vi "PH_Cam_BaseClass.panel.vi"(0 "object ref":refnum<vi>, 5 "error in (no error)":errorcluster) -> (19 "error out":errorcluster)   [LabVIEW 2014, in "PH_Cam_BaseClass.lvlib"]
doc: "This VI is the GUI to control a IEEE1394 Cam.\n\nLicense Agreement for this software:\n\nCopyright (C)\nGesellschaft für Schwerionenforschung, GSI\nPlanckstr. 1\n64291 Darmstadt\nGermany\n\nContact: D.Beck@gsi.de \n\nThis program is free software; you can redistribute it and/or modify it under the terms of the GNU General Public License as published by the Free Software Foundation; either version 2 of the license, or (at your option) any later version.\n\nThis program is distributed in the hope that it will be useful, but WITHOUT ANYW ARRANTY; without even the implied warranty of MERCHANTABILITY or FITNESS FOR A PARTICULAR PURPOSE. See the GNU General License for more details (http://www.gnu.org).\n\nGesellschaft für Schwerionenforschung, GSI\nPlanckstr. 1, 64291 Darmstadt, Germany\nFor all questions and ideas contact: M.Richter@gsi.de, H.Brand@gsi.de or D.Beck@gsi.de.\nLast update: 18-DEC-2002"
uses:
  PH_Cam_BaseClass.lvlib
  PH_StatusHandler/PH_StatusHandler.GUI element.ctl
  PH_Cam_BaseClass.GUI Refs.ctl
  CS_Core/CSObj/CSObj.lvlib
  CS_Core/CSSystem/CSSystemLib/CSSystemLib.lvlib
  PH_Common/PH_Common.lvlib
  PH_Class/PH_Class.lvlib
  PH_StatusHandler/PH_StatusHandler.lvlib
panel:
  out "PSDB Status":u32(colorbox)=6618880 caption="PSDB"
  out "Camera Status":T1 caption="Camera"
  in  "Tab Control":T2(tab)
  in  "Start Cam":bool
  in  "Get Histogram":bool
  in  "Logarithmic":bool
  out "Histogram":u32[](graph)
  in  "Save Image":bool
  in  "Show Image":bool
  in  "Palette":i32(ring) items=["Grey", "Binary", "Gradient", "Rainbow", "Temperature", "HMH"]
  in  "Scale Factor":i32=50 caption="%" min=30 max=500
  in  "Center of Gravity":bool
  in  "Subtract Background":bool
  in  "Center Cross":bool
  in  "Cam List":u32(ring)
  out "Cam Error":errorcluster
  out "Frames per second":dbl(knob) scale=0.0..30.0 scale format="%.1f"
  in  "Get Frame Rate":bool
  in  "Delete":bool
  in  "Exit":bool
  out "loop counter":i32
  # "PCS"
  # "3.40"
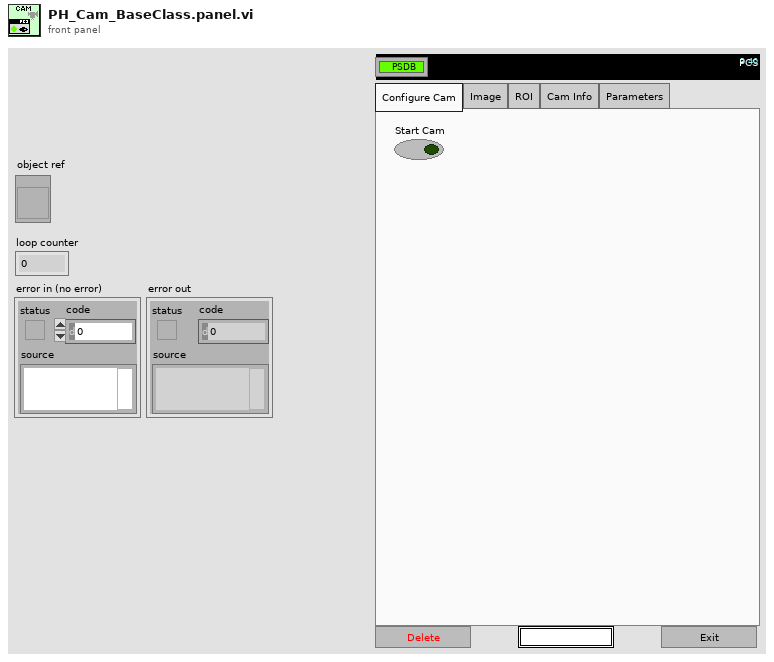
[diagram p1: front panel]
types:
  T1 = typedef "PH_StatusHandler.lvlib/PH_StatusHandler.GUI element.ctl" = u16
  T2 = enum32{"Configure Cam", "Image", "ROI", "Cam Info", "Parameters"}
  T3 = typedef "PH_Cam_BaseClass.lvlib/PH_Cam_BaseClass.GUI Refs.ctl" = cluster{"Frame Rate":refnum<vi>, "Get Frame Rate":refnum<vi>, "Show Image":refnum<vi>, "Get Histogram":refnum<vi>, "Mapping":refnum<vi>, "Histogram":refnum<vi>, "Center Cross":refnum<vi>, "Center of Gravity":refnum<vi>, "Scale Factor [%]":refnum<vi>, "Save Image":refnum<vi>, "Palette":refnum<vi>, "Subtract Background":refnum<vi>, "Cam Error":refnum<vi>, "On":refnum<vi>, "Cam List":refnum<vi>}
  T4 = cluster{"Cam Base ClassGui Refs":T3, "PSDB Status":refnum<vi>, "Status":refnum<vi>}
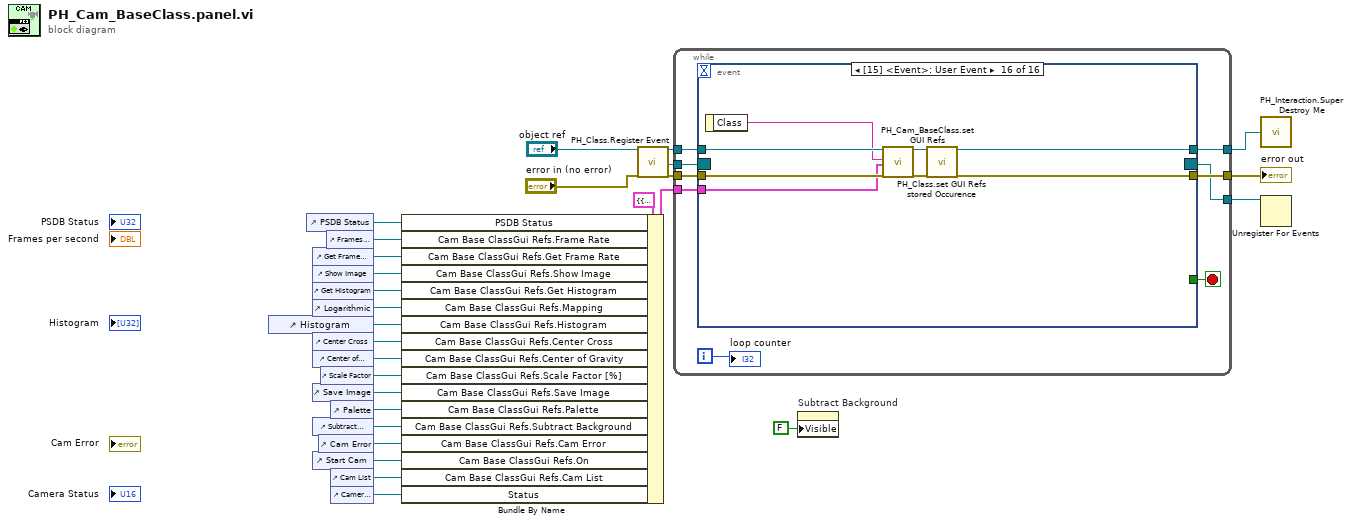
[diagram p0: block diagram]
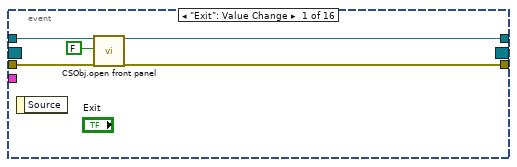
[diagram p2: hidden frame]
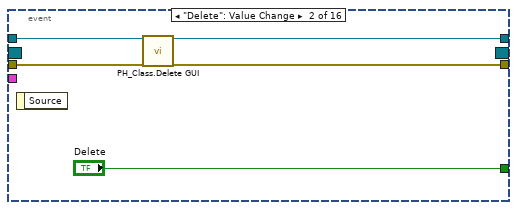
[diagram p3: hidden frame]
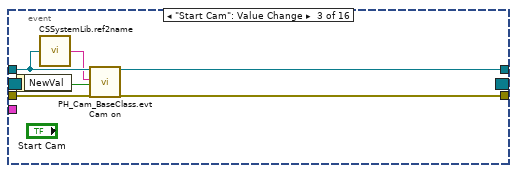
[diagram p4: hidden frame]
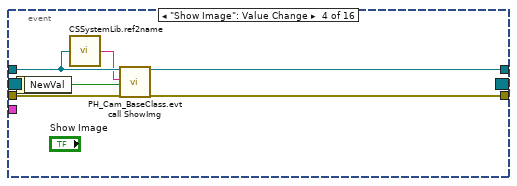
[diagram p5: hidden frame]
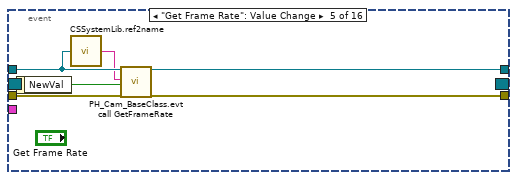
[diagram p6: hidden frame]
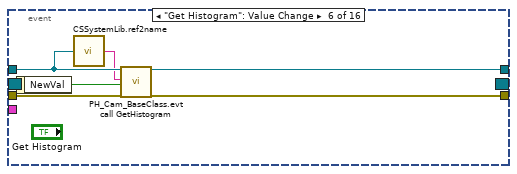
[diagram p7: hidden frame]
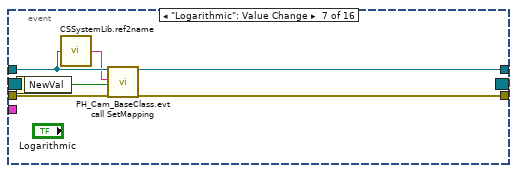
[diagram p8: hidden frame]
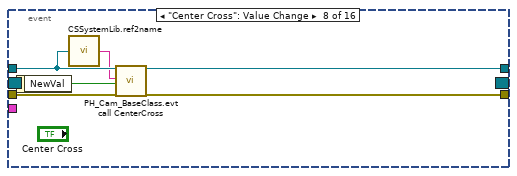
[diagram p9: hidden frame]
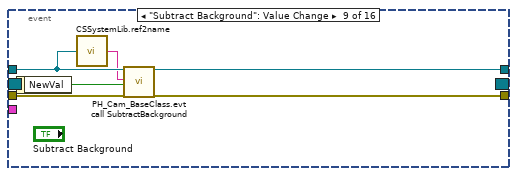
[diagram p10: hidden frame]
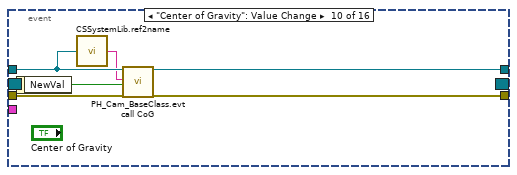
[diagram p11: hidden frame]
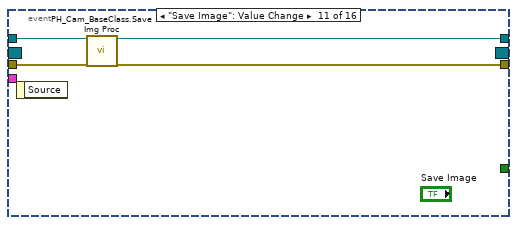
[diagram p12: hidden frame]
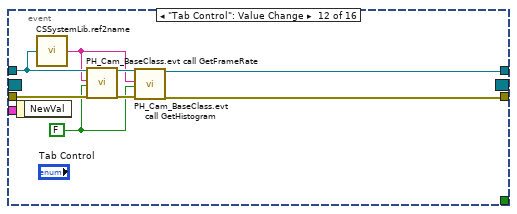
[diagram p13: hidden frame]
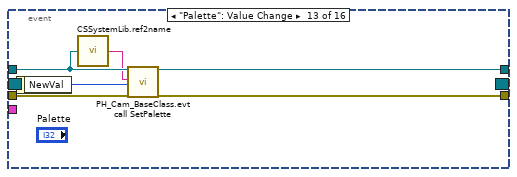
[diagram p14: hidden frame]
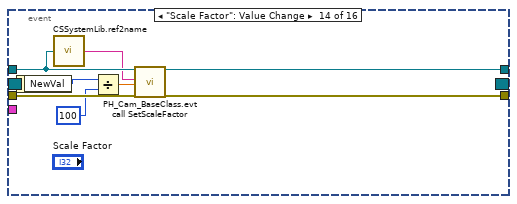
[diagram p15: hidden frame]
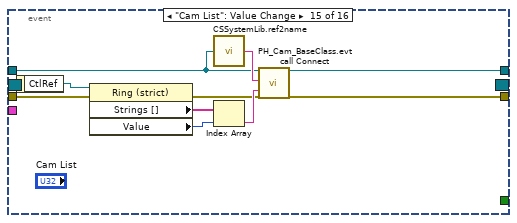
[diagram p16: hidden frame]
diagram:
  n1 = control-ref of="Histogram"() -> (w23:refnum<vi>)
  n2 = control-ref of="PSDB Status"() -> (w4:refnum<vi>)
  n3 = control-ref of="Get Frame Rate"() -> (w27:refnum<vi>)
  n4 = control-ref of="Show Image"() -> (w26:refnum<vi>)
  n5 = control-ref of="Get Histogram"() -> (w25:refnum<vi>)
  n6 = control-ref of="Logarithmic"() -> (w24:refnum<vi>)
  n7 = control-ref of="Center Cross"() -> (w16:refnum<vi>)
  n8 = control-ref of="Center of Gravity"() -> (w19:refnum<vi>)
  n9 = control-ref of="Save Image"() -> (w22:refnum<vi>)
  n10 = control-ref of="Subtract Background"() -> (w15:refnum<vi>)
  n11 = control-ref of="Start Cam"() -> (w12:refnum<vi>)
  n12 = control-ref of="Cam Error"() -> (w13:refnum<vi>)
  n13 = control-ref of="Scale Factor"() -> (w20:refnum<vi>)
  n14 = control-ref of="Frames per second"() -> (w28:refnum<vi>)
  n15 = control-ref of="Palette"() -> (w21:refnum<vi>)
  n16 = control-ref of="Cam List"() -> (w11:refnum<vi>)
  n17 = control-ref of="Camera Status"() -> (w1:refnum<vi>)
  n18 = Bundle By Name(cluster=T4 {"Cam Base ClassGui Refs"={"Frame Rate"=refnum, "Get Frame Rate"=refnum, "Show Image"=refnum, "Get Histogram"=refnum, "Mapping"=refnum, "Histogram"=refnum, "Center Cross"=refnum, "Center of Gravity"=refnum, "Scale Factor [%]"=refnum, "Save Image"=refnum, "Palette"=refnum, "Subtract Background"=refnum, "Cam Error"=refnum, "On"=refnum, "Cam List"=refnum}, "PSDB Status"=refnum, "Status"=refnum} ("GUI Refs to set"), "PSDB Status"=w4, "Cam Base ClassGui Refs.Frame Rate"=w28, "Cam Base ClassGui Refs.Get Frame Rate"=w27, "Cam Base ClassGui Refs.Show Image"=w26, "Cam Base ClassGui Refs.Get Histogram"=w25, "Cam Base ClassGui Refs.Mapping"=w24, "Cam Base ClassGui Refs.Histogram"=w23, "Cam Base ClassGui Refs.Center Cross"=w16, "Cam Base ClassGui Refs.Center of Gravity"=w19, "Cam Base ClassGui Refs.Scale Factor [%]"=w20, "Cam Base ClassGui Refs.Save Image"=w22, "Cam Base ClassGui Refs.Palette"=w21, "Cam Base ClassGui Refs.Subtract Background"=w15, "Cam Base ClassGui Refs.Cam Error"=w13, "Cam Base ClassGui Refs.On"=w12, "Cam Base ClassGui Refs.Cam List"=w11, "Status"=w1) -> (w3:T4)
  n19 = call "PH_Class.Register Event.vi"("i ref in"="object ref", "error in (no error)"="error in (no error)") -> ("i ref out"=w10:refnum<vi>, "Event Registration Refnum"=w8:refnum<event-registration>, "error out"=w9:errorcluster)  [unwired: 15 in]
  n20 = while {
    tunnel: w10 -> [w33]
    tunnel: [w32] -> w17
    tunnel: w9 -> [w35]
    tunnel: [w34] -> w18
    tunnel: w8 -> [w31]
    tunnel: [w30] -> w7
    tunnel: w3 -> [w29]
    i -> [w36]
    stop <- w37 stop-if-true
    n21 = event shown="[15] <Event>: User Event" {
      selector: w31 -> [_ _ _ _ _ _ _ _ _ _ _ _ _ _ _ _]
      dyn-events: [_ _ _ _ _ _ _ _ _ _ _ _ _ _ _ _] -> w30
      timeout: _ -> [_ _ _ _ _ _ _ _ _ _ _ _ _ _ _ _]
      tunnel: [_ "Delete" _ _ _ _ _ _ _ _ _ _ _ _ _ _] -> w37
      tunnel: w33 -> [w42 w46 w52 w56 w62 w68 w74 w80 w86 w92 w99 w102 w110 w118 w126 w139]
      tunnel: w35 -> [w40 w45 w53 w59 w65 w71 w77 w83 w89 w95 w98 w105 w113 w121 w125 w138]
      tunnel: [w39 w43 w48 w58 w64 w70 w76 w82 w88 w94 w96 w103 w111 w119 w123 w133] -> w34
      tunnel: [w38 w44 w49 w57 w63 w69 w75 w81 w87 w93 w97 w106 w112 w120 w124 w135] -> w32
      tunnel: w29 -> [_ _ _ _ _ _ _ _ _ _ _ _ _ _ _ w132]
      event "Exit": Value Change {
        n22 = event-data() -> ()  [unwired: 1 in, 1 out]
        n23 = call "CSObj.open front panel.vi"("i ref in"=w42, "frontPanelOpen"=FALSE ("front panel open"), "error in (no error)"=w40) -> ("i ref out"=w38:refnum<vi>, "error out"=w39:errorcluster)  [unwired: 15 in]
      }
      event "Delete": Value Change {
        n24 = event-data() -> ()  [unwired: 1 in, 1 out]
        n25 = call "PH_Class.Delete GUI.vi"("VI in"=w46, "error in (no error)"=w45) -> ("VI out"=w44:refnum<vi>, "error out"=w43:errorcluster)  [unwired: 16 in]
      }
      event "Start Cam": Value Change {
        n26 = event-data() -> ("NewVal"=w50:bool)  [unwired: 1 in]
        n27 = call "CSSystemLib.ref2name.vi"("obj refnum"=w52) -> ("name"=w51:string)
        n28 = call "PH_Cam_BaseClass.evt Cam on.vi"("i ref in"=w52, "Instance"=w51, "Cam on"=w50, "error in (no error)"=w53) -> ("i ref out"=w49:refnum<vi>, "error out"=w48:errorcluster)  [unwired: 14 in]
      }
      event "Show Image": Value Change {
        n29 = event-data() -> ("NewVal"=w54:bool)  [unwired: 1 in]
        n30 = call "CSSystemLib.ref2name.vi"("obj refnum"=w56) -> ("name"=w55:string)
        n31 = call "PH_Cam_BaseClass.evt call ShowImg.vi"("i ref in"=w56, "Instance"=w55, "Start Cam"=w54, "error in (no error)"=w59) -> ("i ref out"=w57:refnum<vi>, "error out"=w58:errorcluster)  [unwired: 14 in]
      }
      event "Get Frame Rate": Value Change {
        n32 = event-data() -> ("NewVal"=w60:bool)  [unwired: 1 in]
        n33 = call "CSSystemLib.ref2name.vi"("obj refnum"=w62) -> ("name"=w61:string)
        n34 = call "PH_Cam_BaseClass.evt call GetFrameRate.vi"("i ref in"=w62, "Instance"=w61, "Get Frame Rate"=w60, "error in (no error)"=w65) -> ("i ref out"=w63:refnum<vi>, "error out"=w64:errorcluster)  [unwired: 14 in]
      }
      event "Get Histogram": Value Change {
        n35 = event-data() -> ("NewVal"=w66:bool)  [unwired: 1 in]
        n36 = call "CSSystemLib.ref2name.vi"("obj refnum"=w68) -> ("name"=w67:string)
        n37 = call "PH_Cam_BaseClass.evt call GetHistogram.vi"("i ref in"=w68, "Instance"=w67, "Get Histogram"=w66, "error in (no error)"=w71) -> ("i ref out"=w69:refnum<vi>, "error out"=w70:errorcluster)  [unwired: 14 in]
      }
      event "Logarithmic": Value Change {
        n38 = event-data() -> ("NewVal"=w72:bool)  [unwired: 1 in]
        n39 = call "CSSystemLib.ref2name.vi"("obj refnum"=w74) -> ("name"=w73:string)
        n40 = call "PH_Cam_BaseClass.evt call SetMapping.vi"("i ref in"=w74, "Instance"=w73, "Get Histogram"=w72, "error in (no error)"=w77) -> ("i ref out"=w75:refnum<vi>, "error out"=w76:errorcluster)  [unwired: 14 in]
      }
      event "Center Cross": Value Change {
        n41 = event-data() -> ("NewVal"=w78:bool)  [unwired: 1 in]
        n42 = call "CSSystemLib.ref2name.vi"("obj refnum"=w80) -> ("name"=w79:string)
        n43 = call "PH_Cam_BaseClass.evt call CenterCross.vi"("i ref in"=w80, "Instance"=w79, "Center Cross"=w78, "error in (no error)"=w83) -> ("i ref out"=w81:refnum<vi>, "error out"=w82:errorcluster)  [unwired: 14 in]
      }
      event "Subtract Background": Value Change {
        n44 = event-data() -> ("NewVal"=w84:bool)  [unwired: 1 in]
        n45 = call "CSSystemLib.ref2name.vi"("obj refnum"=w86) -> ("name"=w85:string)
        n46 = call "PH_Cam_BaseClass.evt call SubtractBackground.vi"("i ref in"=w86, "Instance"=w85, "Subtract Background"=w84, "error in (no error)"=w89) -> ("i ref out"=w87:refnum<vi>, "error out"=w88:errorcluster)  [unwired: 14 in]
      }
      event "Center of Gravity": Value Change {
        n47 = event-data() -> ("NewVal"=w90:bool)  [unwired: 1 in]
        n48 = call "CSSystemLib.ref2name.vi"("obj refnum"=w92) -> ("name"=w91:string)
        n49 = call "PH_Cam_BaseClass.evt call CoG.vi"("i ref in"=w92, "Instance"=w91, "Set CoG"=w90, "error in (no error)"=w95) -> ("i ref out"=w93:refnum<vi>, "error out"=w94:errorcluster)  [unwired: 14 in]
      }
      event "Save Image": Value Change {
        n50 = event-data() -> ()  [unwired: 1 in, 1 out]
        n51 = call "PH_Cam_BaseClass.Save Img Proc.vi"("VI in"=w99, "error in (no error)"=w98) -> ("VI out"=w97:refnum<vi>, "error out"=w96:errorcluster)  [unwired: 16 in]
      }
      event "Tab Control": Value Change {
        w100 = FALSE
        n52 = event-data() -> ()  [unwired: 1 in, 1 out]
        n53 = call "CSSystemLib.ref2name.vi"("obj refnum"=w102) -> ("name"=w101:string)
        n54 = call "PH_Cam_BaseClass.evt call GetFrameRate.vi"("i ref in"=w102, "Instance"=w101, "Get Frame Rate"=w100, "error in (no error)"=w105) -> ("i ref out"=w107:refnum<vi>, "error out"=w104:errorcluster)  [unwired: 14 in]
        n55 = call "PH_Cam_BaseClass.evt call GetHistogram.vi"("i ref in"=w107, "Instance"=w101, "Get Histogram"=w100, "error in (no error)"=w104) -> ("i ref out"=w106:refnum<vi>, "error out"=w103:errorcluster)  [unwired: 14 in]
      }
      event "Palette": Value Change {
        n56 = event-data() -> ("NewVal"=w108:i32)  [unwired: 1 in]
        n57 = call "CSSystemLib.ref2name.vi"("obj refnum"=w110) -> ("name"=w109:string)
        n58 = call "PH_Cam_BaseClass.evt call SetPalette.vi"("i ref in"=w110, "Instance"=w109, "Palette"=w108, "error in (no error)"=w113) -> ("i ref out"=w112:refnum<vi>, "error out"=w111:errorcluster)  [unwired: 14 in]
      }
      event "Scale Factor": Value Change {
        n59 = event-data() -> ("NewVal"=w115:i32)  [unwired: 1 in]
        n60 = call "CSSystemLib.ref2name.vi"("obj refnum"=w118) -> ("name"=w117:string)
        n61 = Divide(x=w115, y=100) -> (x/y=w114:dbl)
        n62 = call "PH_Cam_BaseClass.evt call SetScaleFactor.vi"("i ref in"=w118, "Instance"=w117, "Scale Factor [%]"=w114, "error in (no error)"=w121) -> ("i ref out"=w120:refnum<vi>, "error out"=w119:errorcluster)  [unwired: 14 in]
      }
      event "Cam List": Value Change {
        n63 = event-data() -> ("CtlRef"=w122:refnum<vi>)  [unwired: 1 in]
        n64 = property class="Ring (strict)"(reference=w122, error in=w125) -> (error out=w127:errorcluster, "Strings []"=w129:string[], "Value"=w130:u32)  [unwired: 1 out]
        n65 = call "CSSystemLib.ref2name.vi"("obj refnum"=w126) -> ("name"=w131:string)
        n66 = Index Array(array=w129, index=w130) -> (element=w128:string)
        n67 = call "PH_Cam_BaseClass.evt call Connect.vi"("i ref in"=w126, "Instance"=w131, "Cam Name"=w128, "error in (no error)"=w127) -> ("i ref out"=w124:refnum<vi>, "error out"=w123:errorcluster)  [unwired: 14 in]
      }
      event User Event {
        n68 = event-data() -> ("Class"=w137:string)  [unwired: 1 in]
        n69 = call "PH_Cam_BaseClass.set GUI Refs.vi"("VI in"=w139, "Class"=w137, "GUI Refs to set"=w132, "error in (no error)"=w138) -> ("VI out"=w136:refnum<vi>, "error out"=w134:errorcluster)  [unwired: 14 in]
        n70 = call "PH_Class.set GUI Refs stored Occurence.vi"("i ref in"=w136, "error in (no error)"=w134) -> ("i ref out"=w135:refnum<vi>, "error out"=w133:errorcluster)  [unwired: 16 in]
      }
    }
    "loop counter" <- w36
  }
  "error out" <- w18
  n71 = property on="Subtract Background" class="Bool (strict)"("Visible"=FALSE) -> ()  [unwired: 2 in, 2 out]
  n72 = call "PH_Interaction.Super Destroy Me.vi"("i ref out"=w17) -> ()
  n73 = Unregister For Events(event registration refnum=w7) -> ()  [unwired: 1 in, 1 out]
